vi "Get Item IO.vi"(8 "error in (no error)":errorcluster, 10 "Item Type":enum16{"RSI Module", "User Variables"}(ring), 11 "Item Ref in":T3 format="%.0x") -> (0 "error out":errorcluster, 1 "Output Data":T9 {"BD Refs"."Data Reference" format="%.0x"}, 2 "Input Data":T6 {"BD Refs"."Data Reference" format="%.0x"}, 3 "Item Ref out":T3 format="%.0x", 4 "Mixed IO":T1, 5 "To FPGA":T2[](array[typedef]) {"VS ref" format="%.0x"}, 7 "From FPGA":T2[](array[typedef]) {"VS ref" format="%.0x"})   [LabVIEW 2020, in "SEECD Engine.lvlib"]
uses:
  SEECD Engine.lvlib
  Type Defs/Data Ref FGV Command.ctl
  <vilib>/NI VeriStand/Custom Device API/Data Reference.ctl
  <vilib>/NI VeriStand/Custom Device API/Custom Device API.lvlib
  <vilib>/NI VeriStand/Custom Device API/Block Data Reference.ctl
  Type Defs/Output Data.ctl
  Type Defs/Input Data.ctl
  <vilib>/NI VeriStand/Custom Device API/Custom Device Item Ref.ctl
  Shared/Type Defs/UDV Data Type.ctl
  Shared/SEECD Shared.lvlib
  Shared/Type Defs/FXP Config.ctl
  Type Defs/UDV Data.ctl
  Type Defs/Mixed IO.ctl
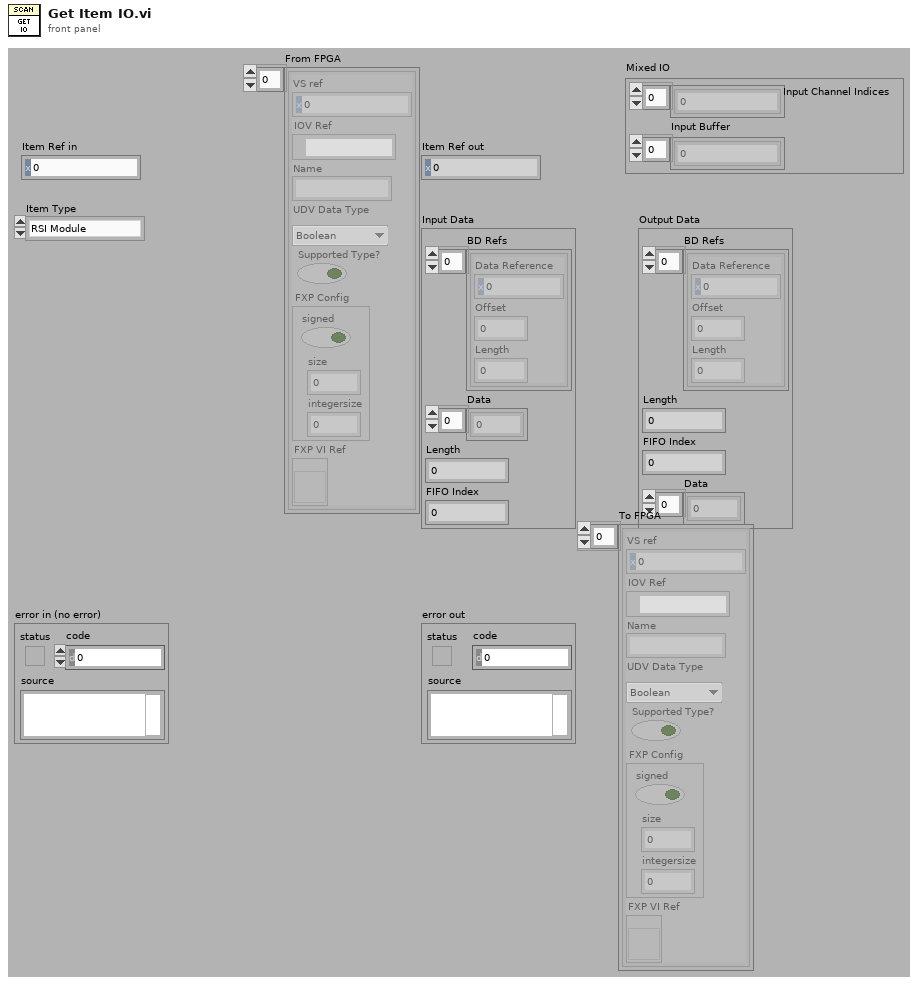
[diagram p1: front panel]
types:
  T1 = typedef "SEECD Engine.lvlib/Mixed IO.ctl" = cluster{"Input Channel Indices":i32[], "Input Buffer":dbl[]}
  T2 = typedef "SEECD Engine.lvlib/UDV Data.ctl" = cluster{"VS ref":T3, "IOV Ref":refnum<k21>, "Name":string, "UDV Data Type":T4, "Supported Type?":bool, "FXP Config":T5, "FXP VI Ref":refnum<vi>}
  T3 = typedef "Custom Device API.lvlib/Custom Device Item Ref.ctl" = u64
  T4 = typedef "SEECD Shared.lvlib/UDV Data Type.ctl" = enum16{"Boolean", "Fixed Point", "Int8", "Int16", "Int32", "Int64", "U32 Bit Field", "UInt8", "UInt16", "UInt32", "UInt64", "Other", "DBL", "SGL"}
  T5 = typedef "SEECD Shared.lvlib/FXP Config.ctl" = cluster{"signed":bool, "size":u32, "integersize":i32}
  T6 = typedef "SEECD Engine.lvlib/Input Data.ctl" = cluster{"BD Refs":T7[], "Data":dbl[], "Length":i32, "FIFO Index":i32}
  T7 = typedef "Custom Device API.lvlib/Block Data Reference.ctl" = cluster{"Data Reference":T8, "Offset":u64, "Length":u64}
  T8 = typedef "Custom Device API.lvlib/Data Reference.ctl" = i32
  T9 = typedef "SEECD Engine.lvlib/Output Data.ctl" = cluster{"BD Refs":T7[], "Length":i32, "FIFO Index":i32, "Data":dbl[]}
  T10 = typedef "SEECD Engine.lvlib/Data Ref FGV Command.ctl" = enum16{"Intialize", "Get", "Update"}
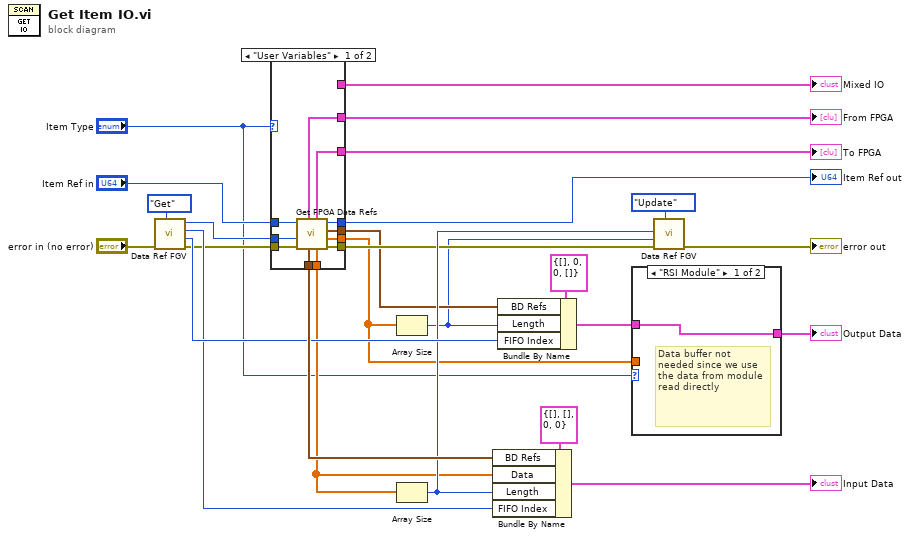
[diagram p0: block diagram]
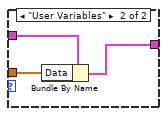
[diagram p2: hidden frame]
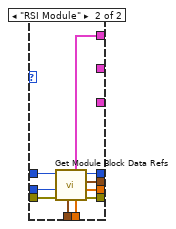
[diagram p3: hidden frame]
diagram:
  n1 = call "Data Ref FGV.vi"("Command"=Data_Ref_FGV_Command."Get", "error in (no error)"="error in (no error)") -> ("error out"=w16:errorcluster, "Output FIFO Index / Length"=w22:i32, "Input FIFO Index / Length"=w21:i32, "Device Ref out"=w11:T3)  [unwired: 6 in]
  n2 = case shown="\"User Variables\"" "Item Type" {
    tunnel: [w33 w47] -> w8
    tunnel: [w34 w46] -> w23
    tunnel: [w32 w45] -> w17
    tunnel: w16 -> [w36 w44]
    tunnel: [w30 w43] -> w14
    tunnel: [w31 w42] -> w1
    tunnel: [w29 w41] -> w13
    tunnel: "Item Ref in" -> [w37 w40]
    tunnel: w11 -> [w35 w39]
    tunnel: [w28 _] -> w7
    tunnel: [w27 _] -> w6
    tunnel: [_ w38] -> w5
    frame "User Variables" {
      n3 = call "Get FPGA Data Refs.vi"("error in"=w36, "Device Ref in"=w35, "Item Ref in"=w37) -> ("error out"=w32:errorcluster, "Output Data"=w31:dbl[], "Output Block Data Refs"=w30:T7[], "Item Ref out"=w29:T3, "Input Data"=w33:dbl[], "To FPGA"=w27:T2[], "Input Block Data Refs"=w34:T7[], "From FPGA"=w28:T2[])  [unwired: 1 in]
    }
    frame "RSI Module" {
      n4 = call "Get Module Block Data Refs.vi"("error in"=w44, "Device Ref in"=w39, "Item Ref in"=w40) -> ("error out"=w45:errorcluster, "Output Data"=w42:dbl[], "Output Block Data Refs"=w43:T7[], "Item Ref out"=w41:T3, "Input Data"=w47:dbl[], "Mixed IO"=w38:T1, "Input Block Data Refs"=w46:T7[])  [unwired: 2 in]
    }
  }
  "Item Ref out" <- w13
  "From FPGA" <- w7
  "To FPGA" <- w6
  "Mixed IO" <- w5
  n5 = Array Size(array=w1) -> (size(s)=w9:i32)
  n6 = Array Size(array=w8) -> (size(s)=w20:i32)
  n7 = Bundle By Name(cluster=T6 {"BD Refs"=[], "Data"=[], "Length"=0, "FIFO Index"=0} ("Input Data"), "BD Refs"=w23, "Data"=w8, "Length"=w20, "FIFO Index"=w21) -> (→"Input Data":T6)
  n8 = Bundle By Name(cluster=T9 {"BD Refs"=[], "Length"=0, "FIFO Index"=0, "Data"=[]} ("Output Data"), "BD Refs"=w14, "Length"=w9, "FIFO Index"=w22) -> (w3:T9)
  n9 = case shown="\"RSI Module\"" "Item Type" {
    tunnel: w3 -> [w48 w51]
    tunnel: [w48 w50] -> w2
    tunnel: w1 -> [_ w49]
    frame "RSI Module" {
      # "Data buffer not needed since we use the data from module read directly"
    }
    frame "User Variables" {
      n10 = Bundle By Name(cluster=w51, "Data"=w49) -> (w50:T9)
    }
  }
  "Output Data" <- w2
  n11 = call "Data Ref FGV.vi"("Command"=Data_Ref_FGV_Command."Update", "error in (no error)"=w17, "Output Length"=w9, "Input Length"=w20) -> ("error out"=→"error out":errorcluster)  [unwired: 4 in, 3 out]
